vi "Preview.vi"(6 "timeout in ms (-1)":i32, 8 "error in (no error)":errorcluster, 11 "queue in":refnum<queue>) -> (0 "error out":errorcluster, 1 "Data":variant, 2 "Command":string, 3 "queue out":refnum<queue>, 4 "timed out?":bool)   [LabVIEW 2013, in "命令队列.lvlib"]
uses:
  Command.ctl
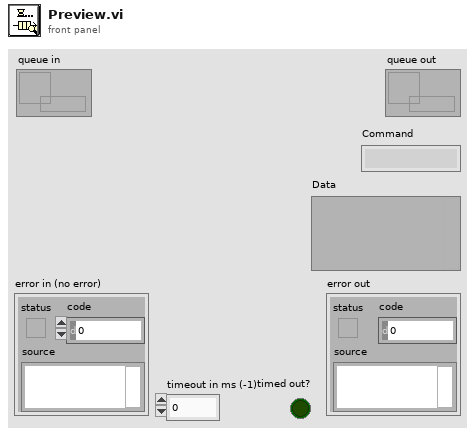
[diagram p1: front panel]
types:
  T1 = typedef "命令队列.lvlib/Command.ctl" = cluster{"command":string, "data":variant}
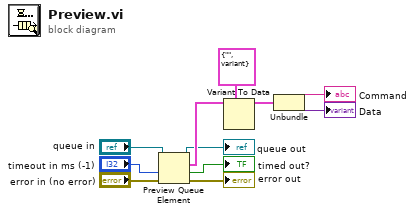
[diagram p0: block diagram]
diagram:
  n1 = Preview Queue Element(queue="queue in", timeout in ms (-1)="timeout in ms (-1)", error in (no error)="error in (no error)") -> (queue out=→"queue out":refnum<queue>, element=w8:cluster{"command":string, "data":variant}, timed out?=→"timed out?":bool, error out=→"error out":errorcluster)
  n2 = Variant To Data(type=T1 {"command"="", "data"=variant} ("command queue element"), Variant=w8) -> (data=w9:T1)  [unwired: 1 in, 1 out]
  n3 = Unbundle(w9) -> ("command"=→"Command":string, "data"=→"Data":variant)
